vi "Untitled 1.vi"() -> ()   [LabVIEW 2025]
uses:
  <vilib>/Serenial/G Augmented-Reality Toolkit/g_ar_toolkit.examples/g_ar_toolkit.examples.lvlib
panel:
  out "Numeric 3":dbl
  in  "Numeric 2":dbl
  in  "Numeric":dbl
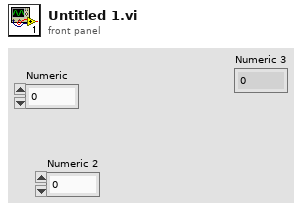
[diagram p1: front panel]
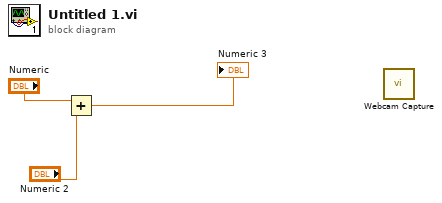
[diagram p0: block diagram]
diagram:
  n1 = Add(x="Numeric", y="Numeric 2") -> (x+y=→"Numeric 3":dbl)
  n2 = call <vilib>:"Webcam Capture.vi"() -> ()  [unwired: 12 in]
